vi "CleanUp.vi"(0 "class data in":refnum<class "SceneObject.lvclass">, 5 "error in":errorcluster) -> (14 "class data out":refnum<class "SceneObject.lvclass">, 19 "error out":errorcluster)   [LabVIEW 2010, in "RenderBase.lvlib" / "SceneObject.lvclass"]
doc: "Closes open references."
uses:
  SceneObject.lvclass
  SceneObject.lvclass/SceneObject.ctl
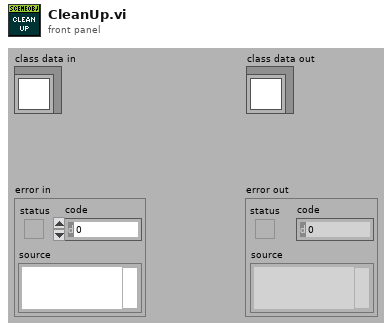
[diagram p1: front panel]
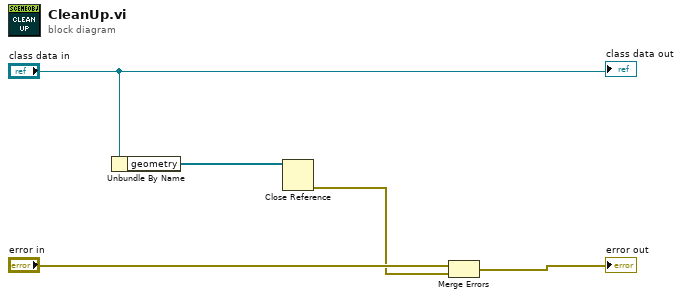
[diagram p0: block diagram]
diagram:
  n1 = Unbundle By Name("class data in") -> ("geometry"=w1:refnum<vi>[])
  n2 = Close Reference(reference=w1) -> (error out=w3:errorcluster)  [unwired: 1 in]
  n3 = Merge Errors("error in", w3) -> (→"error out":errorcluster)
  "class data out" <- "class data in"
